vi "bgk_data_acquisition_loop_02_01.vi"(7 "Period (s)":dbl=600.0 caption="采样周期 (s)" format="%#_13g", 8 "error in (no error)":errorcluster caption="错误输入（无错误）", 11 "Message Queues":T1 caption="消息队列") -> (0 "error out":errorcluster caption="错误输出")   [LabVIEW 2015]
uses:
  message_queue/all_rt_message_queues.ctl
  message_queue/message_cluster.ctl
  <vilib>/Platform/TimedLoop/XDataNode/timing_clust.ctl
  <vilib>/Platform/TimedLoop/XDataNode/nitl_modes.ctl
  <vilib>/Platform/TimedLoop/XDataNode/wakeup.ctl
  <vilib>/Platform/TimedLoop/XDataNode/loadnilvce.vi
  <vilib>/Instr/_visa.llb/VISA Configure Serial Port (Instr).vi
  globals/global_all_rt_loop_stop.vi
  <vilib>/Platform/TimedLoop/XDataNode/XDataNode.xnode
  <vilib>/Platform/TimedLoop/XDataNode/XDNodeRunTimeDep.lvlib
  message_queue/message_queue.lvlib
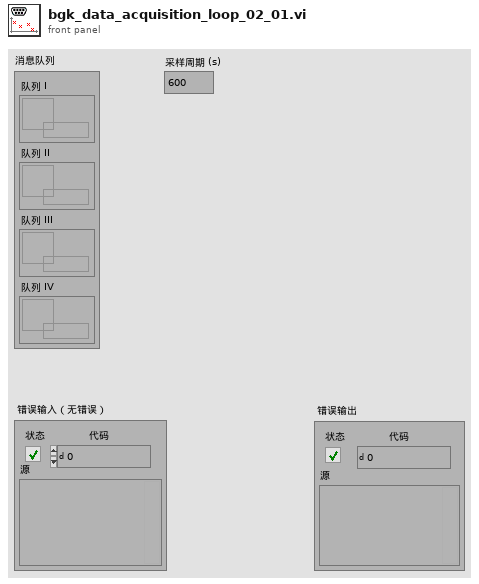
[diagram p1: front panel]
types:
  T1 = typedef "message_queue.lvlib/all_rt_message_queues.ctl" = cluster{"Queue I":refnum<queue>, "Queue II":refnum<queue>, "Queue III":refnum<queue>, "Queue IV":refnum<queue>}
  T2 = typedef "XDNodeRunTimeDep.lvlib/timing_clust.ctl" = cluster{"Expected End [f-1]":u64, "Actual End [f-1]":u64, "Finished Late? [f-1]":bool, "Expected End [i-1]":u64, "Actual End [i-1]":u64, "Finished Late? [i-1]":bool, "Expected Start [i]":u64, "Actual Start [i]":u64, "Expected Start [f]":u64, "Actual Start [f]":u64, "Source Name":string, "Structure Name":string, "Period":i64, "Deadline":i64, "Offset":i64, "Start":i64, "Priority":i32, "Timeout":i32, "Mode":T3, "Wakeup Reason":T4, "Error":errorcluster, "Source Type":string, "Secondary Source Type":string, "Global End Time":u64, "Global Start Time":u64, "Frame Duration":u64, "Iteration Duration":u64, "Assigned CPU":i32, "I/O Scan Engine Mode":u32}
  T3 = typedef "XDNodeRunTimeDep.lvlib/nitl_modes.ctl" = enum32{"No Change", "Process missed periods, maintain original phase", "Discard missed periods, maintain original phase", "Process missed periods, ignore original phase", "Discard missed periods, ignore original phase"}
  T4 = typedef "XDNodeRunTimeDep.lvlib/wakeup.ctl" = enum32{"Normal", "Aborted", "Asynchronous wakeup", "Timing source error", "Timed loop error", "Timeout"}
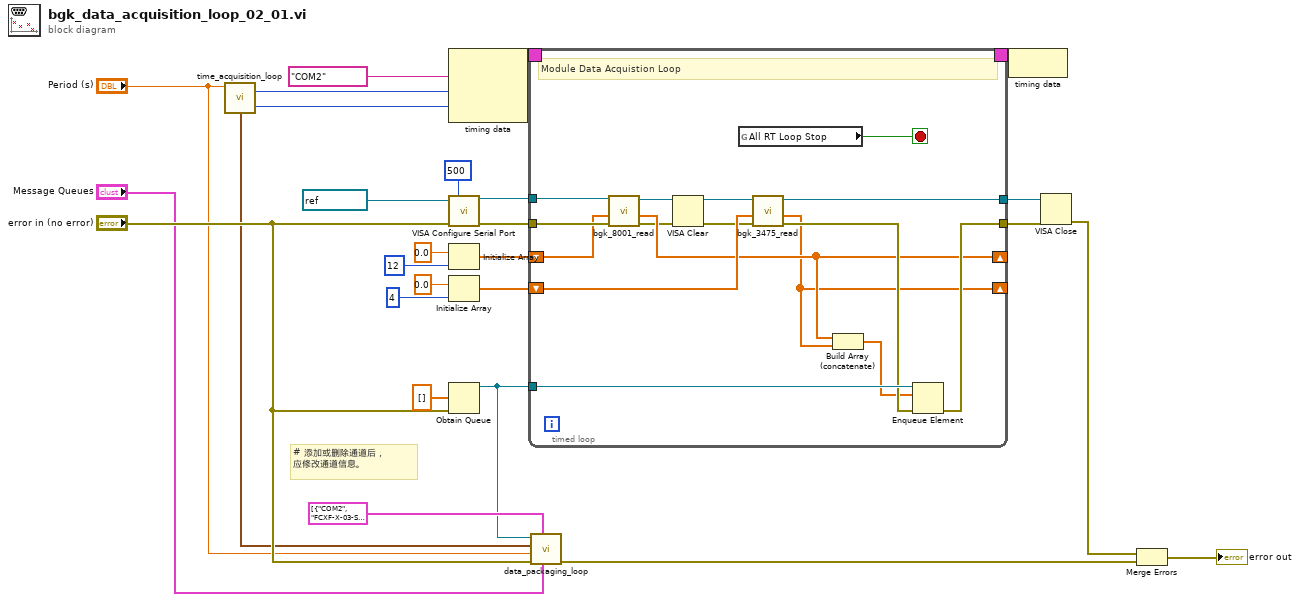
[diagram p0: block diagram]
diagram:
  # "# 添加或删除通道后，\n应修改通道信息。"
  n1 = call "time_acquisition_loop.vi"("Period (s)"="Period (s)") -> ("t0 (scan)"=w1:i64, "Period (scan)"=w2:i64, "timestamp output"=w4:timestamp)  [unwired: 4 in]
  n2 = node-c288("COM2" ("Structure Name"), w2, w1) -> (w26:T2)
  n3 = call-poly "VISA Configure Serial Port"("VISA resource name"=refnum<visa-resource-name> "COM2", "timeout (10sec)"=u32 500, "error in (no error)"="error in (no error)") -> ("VISA resource name out"=w19:refnum<visa-resource-name>, "error out"=w23:errorcluster)  [unwired: 11 in]
  n4 = Initialize Array(0.0 ("元素"), 12 ("维数大小")) -> (w10:dbl[])
  n5 = Initialize Array(0.0 ("元素"), 4 ("维数大小")) -> (w6:dbl[])
  n6 = Obtain Queue(element data type=dbl[] [] ("数据类型"), error in (no error)="error in (no error)") -> (queue out=w12:refnum<queue>)  [unwired: 3 in, 2 out]
  n7 = timed-loop {
    timing: w26 -> [_]
    timing-out: [_] -> w25
    tunnel: w12 -> [w42]
    tunnel: w23 -> [w35]
    tunnel: [w41] -> w21
    tunnel: [w39] -> w22
    tunnel: w19 -> [w36]
    shift-right: [w32] -> _
    shift-left: w10 -> [w34]
    shift-right: [w31] -> _
    shift-left: w6 -> [w33]
    stop <- w43 stop-if-true
    # "Module Data Acquistion Loop"
    n8 = call "bgk_8001_read.vi"("error in (no error)"=w35, "Last Data Array"=w34, "VISA Ref Input"=w36) -> ("error out"=w29:errorcluster, "New Data Array"=w32:dbl[], "VISA Ref Output"=w40:refnum<visa-resource-name>)  [unwired: 6 in]
    n9 = VISA Clear(VISA resource name=w40, error in (no error)=w29) -> (VISA resource name out=w30:refnum<visa-resource-name>, error out=w28:errorcluster)
    n10 = global read "global_all_rt_loop_stop.vi" "All RT Loop Stop"() -> (w43:bool)
    n11 = call "bgk_3475_read.vi"("error in (no error)"=w28, "Last Data Array"=w33, "VISA Ref Input"=w30) -> ("error out"=w38:errorcluster, "New Data Array"=w31:dbl[], "VISA Ref Output"=w39:refnum<visa-resource-name>)  [unwired: 6 in]
    n12 = Build Array (concatenate)(w32, w31) -> (w37:dbl[])
    n13 = Enqueue Element(queue=w42, element=w37, error in (no error)=w38) -> (error out=w41:errorcluster)  [unwired: 1 in, 2 out]
  }
  n14 = call "data_packaging_loop.vi"("Message Queues"="Message Queues", "channel info array"=cluster{"Module":string, "Channel":string}[] [{"Module"="COM2", "Channel"="FCXF-X-03-S07"}, {"Module"="COM2", "Channel"="FCXF-X-03-T07"}, {"Module"="COM2", "Channel"="FCXF-X-03-S08"}, {"Module"="COM2", "Channel"="FCXF-X-03-T08"}, {"Module"="COM2", "Channel"="FCXF-X-03-S09"}, {"Module"="COM2", "Channel"="FCXF-X-03-T09"}, {"Module"="COM2", "Channel"="FCXF-X-03-S10"}, {"Module"="COM2", "Channel"="FCXF-X-03-T10"}, {"Module"="COM2", "Channel"="FCXF-X-01-D02"}, {"Module"="COM2", "Channel"="FCXF-X-01-T01"}, {"Module"="COM2", "Channel"="FCXF-X-05-D01"}, {"Module"="COM2", "Channel"="FCXF-X-05-T01"}, {"Module"="COM2", "Channel"="FCXF-X-01-D01"}, {"Module"="COM2", "Channel"="FCXF-X-02-D01"}, {"Module"="COM2", "Channel"="FCXL-X-03-D01"}, {"Module"="COM2", "Channel"="FCXF-X-04-D01"}], "error in (no error)"="error in (no error)", "sampling period (s)"="Period (s)", "timestamp"=w4, "data queue"=w12) -> ("error out"=w15:errorcluster)  [unwired: 5 in]
  n15 = node-c288(w25) -> ()
  n16 = VISA Close(VISA resource name=w22, error in (no error)=w21) -> (error out=w20:errorcluster)
  n17 = Merge Errors(w20, w15) -> (→"error out":errorcluster)
